vi "ProcessVirtualChannels.vi"(8 "error in (no error)":errorcluster, 11 "tdms ref in":refnum<k34>) -> (0 "error out":errorcluster, 3 "tdms ref out":refnum<k34>)   [LabVIEW 2017, in "DataExplorerSupport.lvlib"]
uses:
  <vilib>/addons/InsightCM/Utilities/DataExplorerSupport/DataExplorerSupport.lvlib
  <vilib>/addons/InsightCM/Utilities/Tdms/Tdms.lvlib
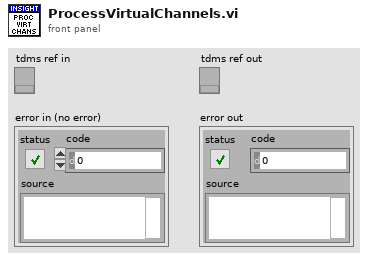
[diagram p1: front panel]
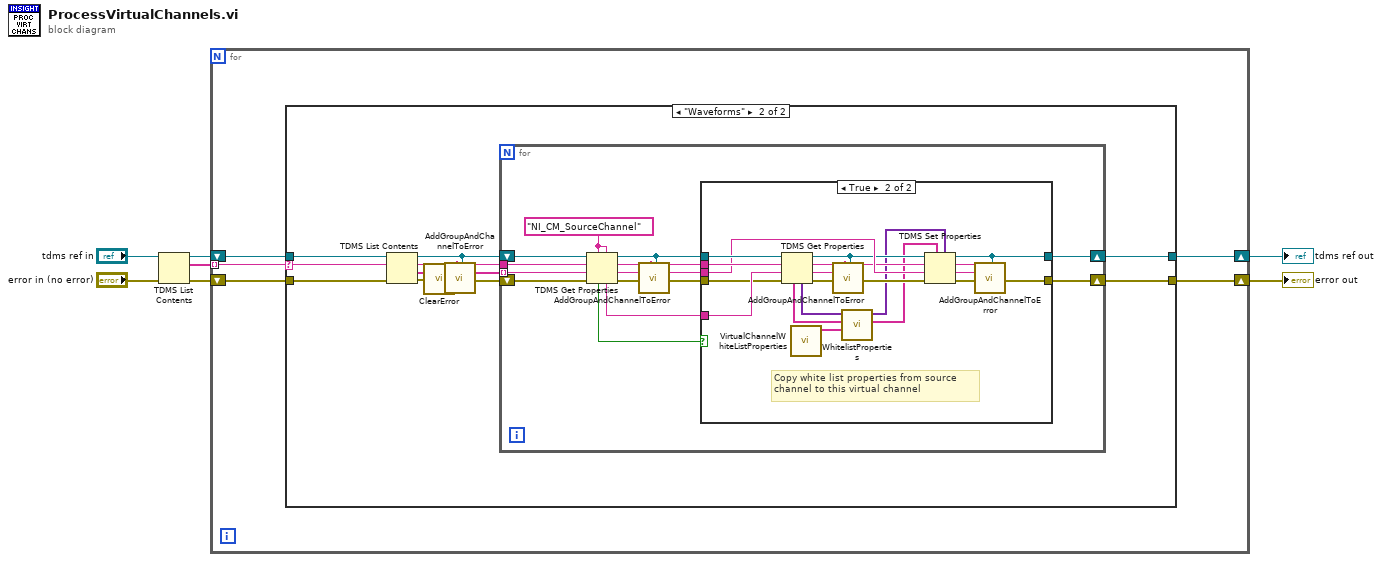
[diagram p0: block diagram]
diagram:
  n1 = TDMS List Contents(4:"error in (no error)", 7:"tdms ref in") -> (0:w2:errorcluster, 2:w1:string[], 3:w4:refnum<k34>)  [unwired: 1 in, 1 out]
  n2 = for {
    shift-right: [w11] -> w6
    shift-left: w4 -> [w10]
    shift-right: [w12] -> w7
    shift-left: w2 -> [w9]
    tunnel: w1 -> [w8] mode=indexing
    n3 = case shown="\"Waveforms\"" w8 {
      selector: w8 -> [_ w15]
      tunnel: [w13 w25] -> w12
      tunnel: [w14 w20] -> w11
      tunnel: w10 -> [w14 w17]
      tunnel: w9 -> [w13 w16]
      frame Default {
      }
      frame "Waveforms" {
        n4 = TDMS List Contents(4:w16, 6:w15, 7:w17) -> (0:w18:errorcluster, 1:w19:string[], 2:w23:string, 3:w24:refnum<k34>)
        n5 = call <vilib>:"ClearError.vi"("error in (no error)"=w18) -> ("error out"=w21:errorcluster)
        n6 = call <vilib>:"AddGroupAndChannelToError.vi"("error in (no error)"=w21, "group name in"=w23, "Refnum in"=w24) -> ("error out"=w22:errorcluster)  [unwired: 16 in]
        n7 = for {
          tunnel: w19 -> [w37] mode=indexing
          tunnel: w23 -> [w38]
          shift-right: [w27] -> w25
          shift-left: w22 -> [w36]
          shift-right: [w26] -> w20
          shift-left: w24 -> [w39]
          w35 = "NI_CM_SourceChannel" ("property name")
          n8 = TDMS Get Properties(5:w35, 7:w35, 8:w36, 9:w37, 10:w38, 11:w39) -> (0:w34:errorcluster, 1:w28:string, 2:w29:string, 3:w30:refnum<k34>, 4:w32:string, 6:w33:bool)
          n9 = call <vilib>:"AddGroupAndChannelToError.vi"("error in (no error)"=w34, "channel name in"=w28, "group name in"=w29, "Refnum in"=w30) -> ("error out"=w31:errorcluster)  [unwired: 15 in]
          n10 = case shown="True" w33 {
            tunnel: w32 -> [_ w59]
            tunnel: w31 -> [w41 w57]
            tunnel: w30 -> [w40 w61]
            tunnel: w29 -> [_ w60]
            tunnel: w28 -> [_ w58]
            tunnel: [w41 w50] -> w27
            tunnel: [w40 w47] -> w26
            frame False {
            }
            frame True {
              # "Copy white list properties from source \nchannel to this virtual channel"
              n11 = TDMS Get Properties(8:w57, 9:w59, 10:w60, 11:w61) -> (0:w56:errorcluster, 1:w54:string, 2:w52:string, 3:w53:refnum<k34>, 4:w44:variant[], 6:w45:string[])  [unwired: 2 in]
              n12 = call <vilib>:"VirtualChannelWhiteListProperties.vi"() -> ("virtual channel white list properties"=w46:string[])  [unwired: 11 in]
              n13 = call <vilib>:"AddGroupAndChannelToError.vi"("error in (no error)"=w56, "channel name in"=w54, "group name in"=w52, "Refnum in"=w53) -> ("error out"=w55:errorcluster)  [unwired: 15 in]
              n14 = call <vilib>:"WhitelistProperties.vi"("white list property names"=w46, "property names in"=w45, "property values in"=w44) -> ("property names out"=w42:string[], "property values out"=w43:variant[])  [unwired: 7 in]
              n15 = TDMS Set Properties(5:w43, 7:w42, 8:w55, 9:w58, 10:w52, 11:w53) -> (0:w51:errorcluster, 1:w48:string, 2:w49:string, 3:w47:refnum<k34>)
              n16 = call <vilib>:"AddGroupAndChannelToError.vi"("error in (no error)"=w51, "channel name in"=w48, "group name in"=w49, "Refnum in"=w47) -> ("error out"=w50:errorcluster)  [unwired: 15 in]
            }
          }
        }
      }
    }
  }
  "error out" <- w7
  "tdms ref out" <- w6
